vi "target.vi"   [LabVIEW 2020]
uses:
  <vilib>/rvi/DataTransferAndStorage/Container/XNode/niFpgaContainer.xnode
  <vilib>/rvi/interface/RandomDataEmulation/nirviRandomDataFpgaReadWriteTemplate.vi
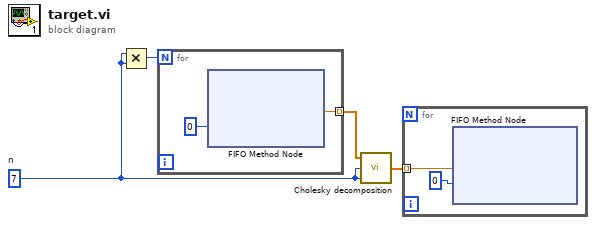
[diagram p0: block diagram]
diagram:
  w2 = 7  # n
  n1 = Multiply(x=w2, y=w2) -> (x*y=w1:i32)
  n2 = for {
    N: w1 -> [_]
    tunnel: [w6] -> w4 mode=indexing
    n3 = xnode ("FIFO Method Node")("Timeout"=0) -> ("Element"=w6:sgl)  [unwired: 1 in, 2 out]
  }
  n4 = call "Cholesky decomposition.vi"("n"=w2, "m"=w2, "A"=w4) -> ("L"=w3:sgl[])
  n5 = for {
    tunnel: w3 -> [w7] mode=indexing
    n6 = xnode ("FIFO Method Node")("Element"=w7, "Timeout"=0) -> ()  [unwired: 1 in, 2 out]
  }
